vi "Magmapper_Tim.vi"() -> ()   [LabVIEW 2020]
uses:
  Labview_dependencies/locked.vi
  Labview_dependencies/haltnow.vi
  <vilib>/Analysis/NI_AALBase.lvlib
panel:
  out "Lock state":bool
  in  "Centering steps":dbl[](array[numeric])
  in  "Start centering":bool
  in  "Theta abs":dbl
  out "Theta pos":dbl
  in  "Initialisation Theta commands":string[](array[string])=["BASE($$$AXIS$$$)", "BACKLASH(OFF)", "ATYPE=43", "UNITS=16*32", "SPEED=1", "CREEP=.1", "FASTDEC=1", "ACCEL=1", "DECEL=1", "DEFPOS(0)", "WDOG=ON", "BASE(0)"]
  in  "Theta Step":dbl
  in  "Theta End":dbl
  in  "Theta Start":dbl
  out "Theta axis on":bool=TRUE
  in  "Theta rel":dbl
  in  "Z Step":dbl
  in  "Z End":dbl
  in  "Z Start":dbl
  in  "Y Step":dbl
  in  "Y End":dbl
  in  "Y Start":dbl
  in  "X Step":dbl
  in  "X End":dbl
  in  "X Start":dbl
  in  "Clear buffers":bool
  in  "Initialisation XYZ commands":string[](array[string])=["BASE($$$AXIS$$$)", "BACKLASH(OFF)", "ATYPE=43", "UNITS=2560", "SPEED=10", "CREEP=5", "FASTDEC=100", "ACCEL=10", "DECEL=10", "DATUM_IN=$$$AXIS$$$+5", "FS_LIMIT = REP_DIST + 10", "RS_LIMIT = -REP_DIST - 10", "WDOG=ON", "DATUM($$$DATUM$$$)", "ALT_WAIT", "FS_LIMIT=$$$FS$$$", "RS_LIMIT=$$$RS$$$", "BASE(0)"]
  in  "Read grid":bool
  in  "Filename for grid readings":path
  in  "Slope (b)":dbl=1.14189
  in  "Intercept (a)":dbl=-0.010254
  out "message":string="Error messages might appear here."
  in  "Initialise":bool
  in  "Stop movement":bool
  out "Z pos":dbl
  out "Y pos":dbl
  out "X pos":dbl
  in  "Move relative":bool
  in  "Move absolute":bool
  in  "Z rel":dbl
  in  "Y rel":dbl
  in  "X rel":dbl
  in  "Z abs":dbl
  in  "Y abs":dbl
  in  "X abs":dbl
  # "Set field-vs-voltage relationship (B = a + bV)"
  # "Current position"
  # "Move to absolute position"
  # "Move to relative position"
  # "Note: STOP is not yet implemented.\nEither manually stop the VI running \n(usual stop button below menu bar)\nor if urgent turn off the power to the \nmagnet  mapper (red rocker switch)."
  # "Read over grid"
  # "Note: Circular axis should be set  on or off before running the VI, and may not be changed while running."
  # "Greyed items are disabled (not yet implemented)."
  # "List of initialisation commands to feed to the MC 405 controller.  Use ALT_WAIT instead of WAIT IDLE to avoid timeouts.  Commands will be run for each (X,Y,Z) axis, replacing $$$AXIS$$$ with the actual axis, $$$DATUM$$$ with the corresponding datum method, $$$FS$$$ and $$$RS$$$ with the corrsponding limits, each time.   If you change the commands and want to keep them when you close the VI, remember to select the array (whole thing, not just index or individual elements), right click, Data operations, Make Current Value Default."
  # "Move near centre by eye then push start"
  # "Minimum step size is 0.05mm. Micro-stepping down to 0.00625mm is possible but not reccommendded as it not necessarily accurate and may cause excess movement during grid reading"
  # "List of initialisation commands to feed to the MC 405 controller.  Use ALT_WAIT instead of WAIT IDLE to avoid timeouts.  Commands will be run for the Theta axis, replacing $$$AXIS$$$ with the actual axis.   If you change the commands and want to keep them when you close the VI, remember to select the array (whole thing, not just index or individual elements), right click, Data operations, Make Current Value Default."
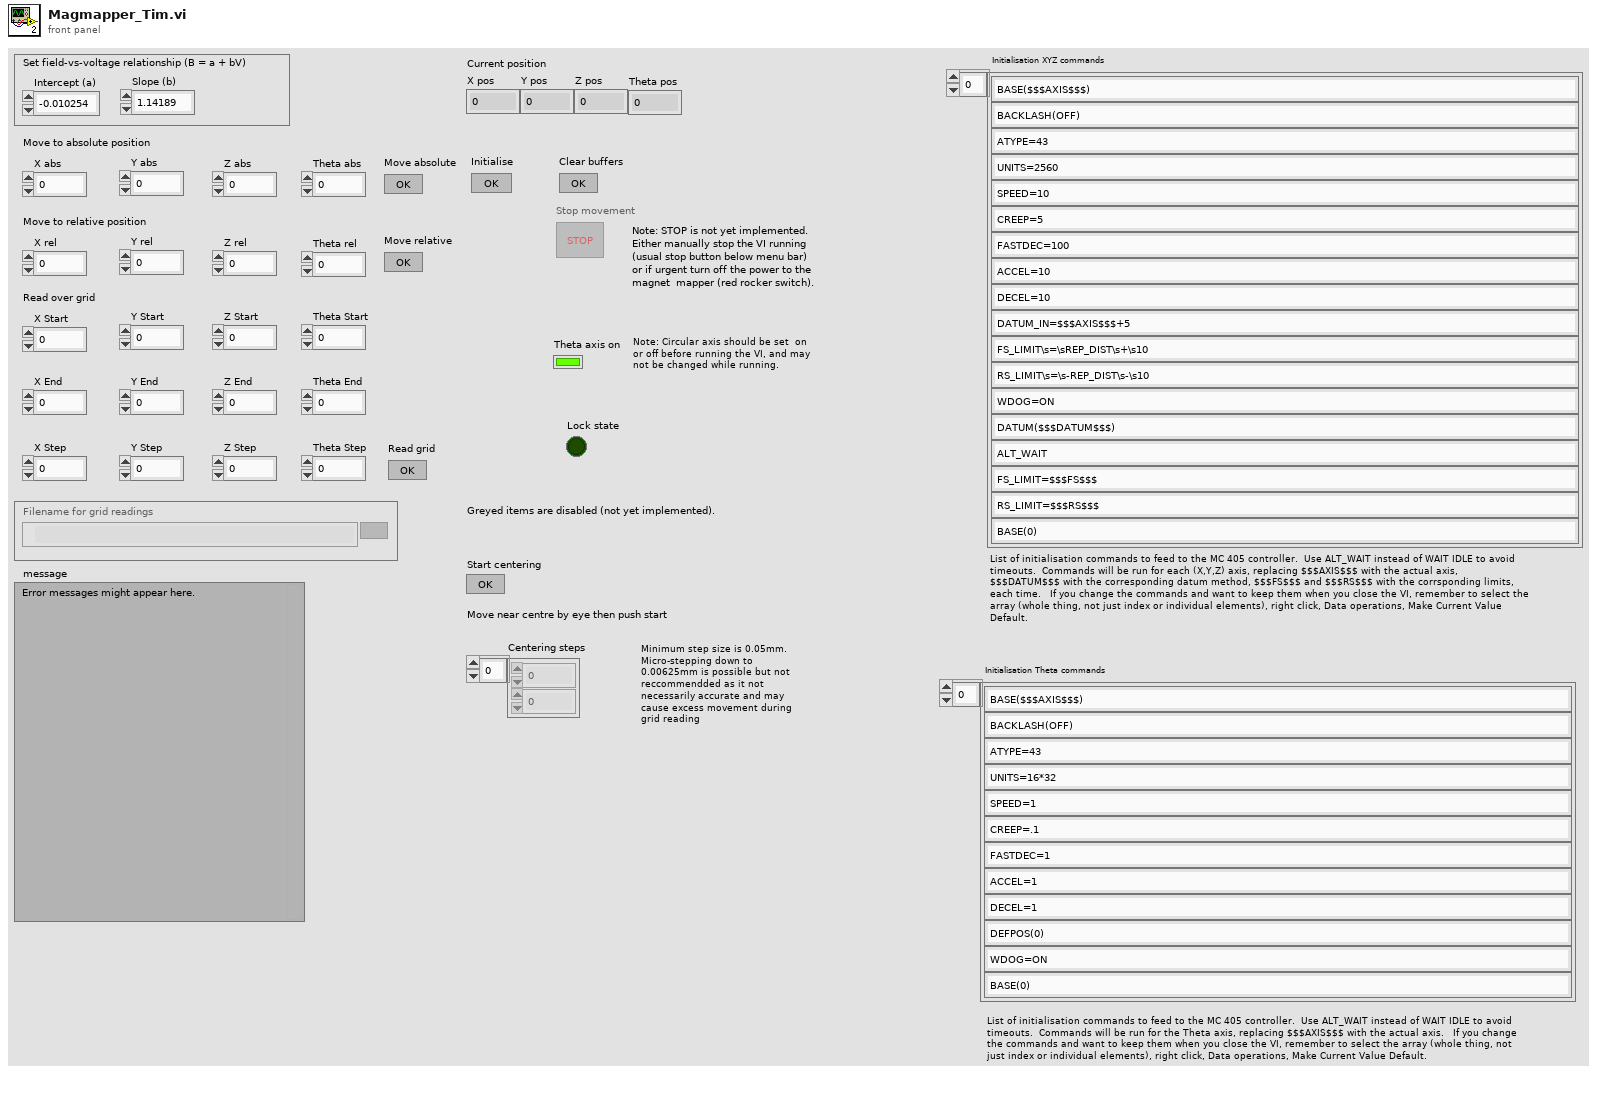
[diagram p1: front panel]
types:
  T1 = enum16{"open", "replace", "create", "open or create", "replace or create", "replace or create with confirmation"}
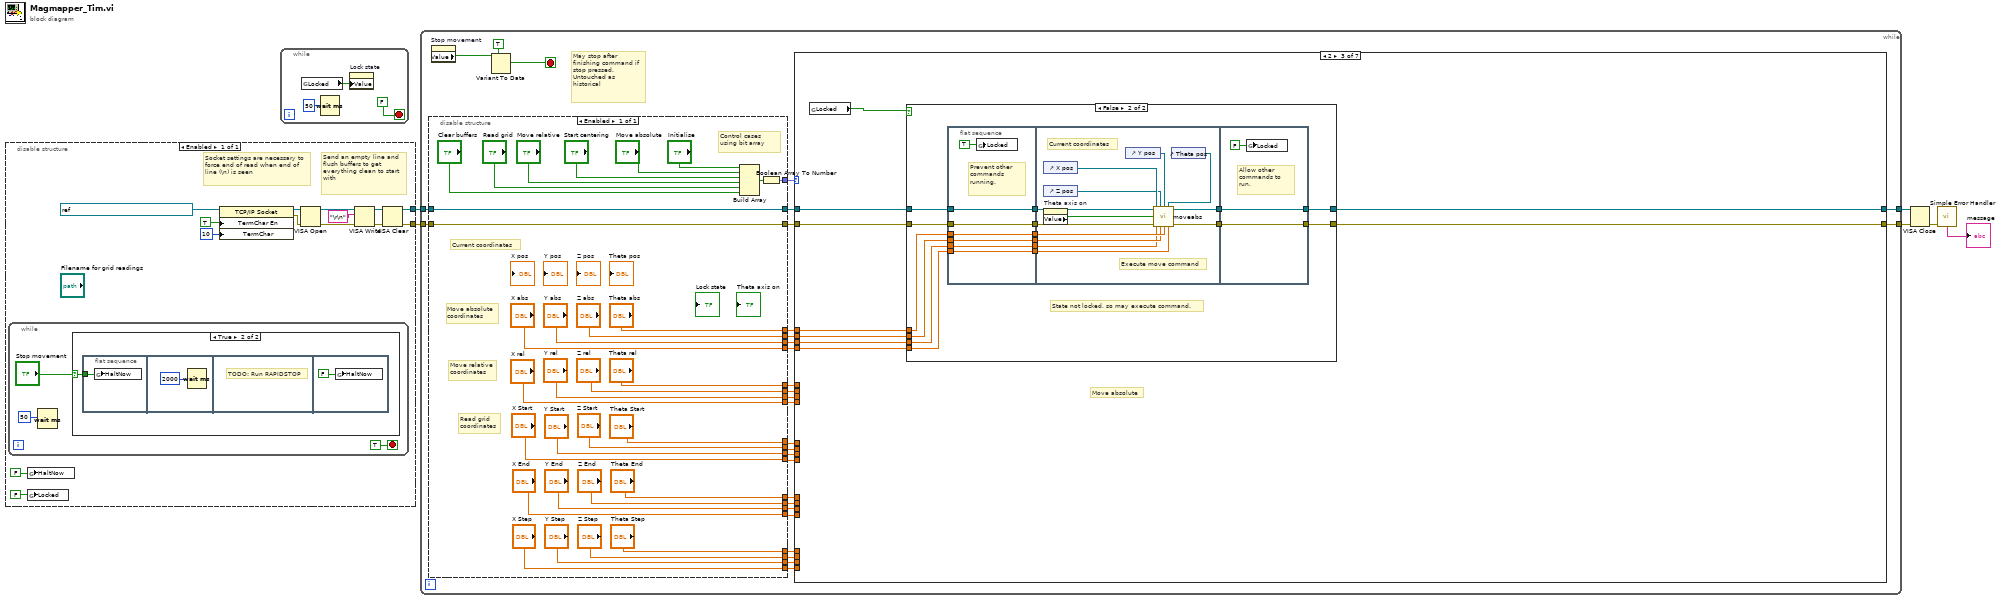
[diagram p0: block diagram]
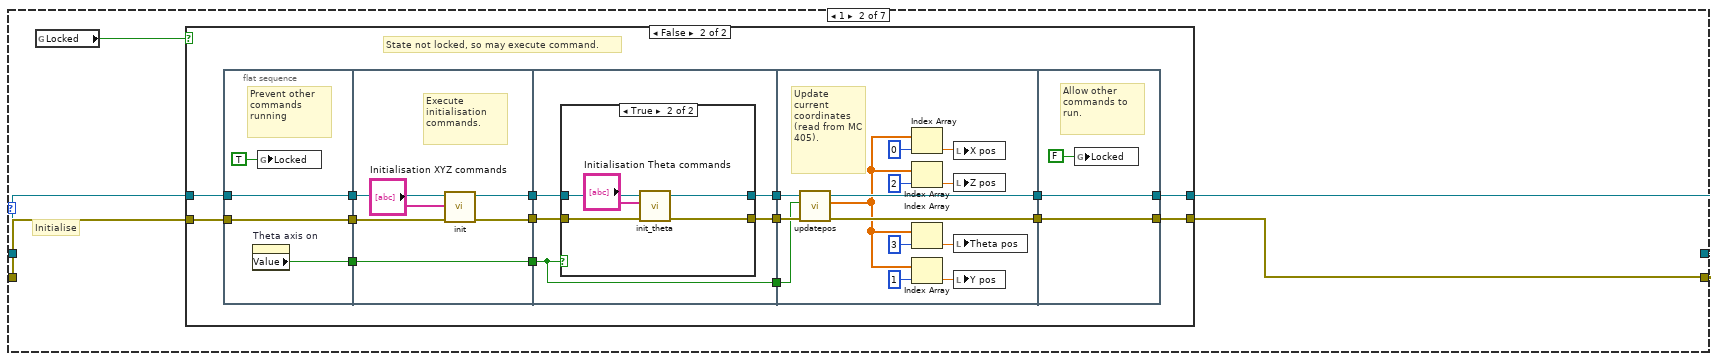
[diagram p4: hidden frame]
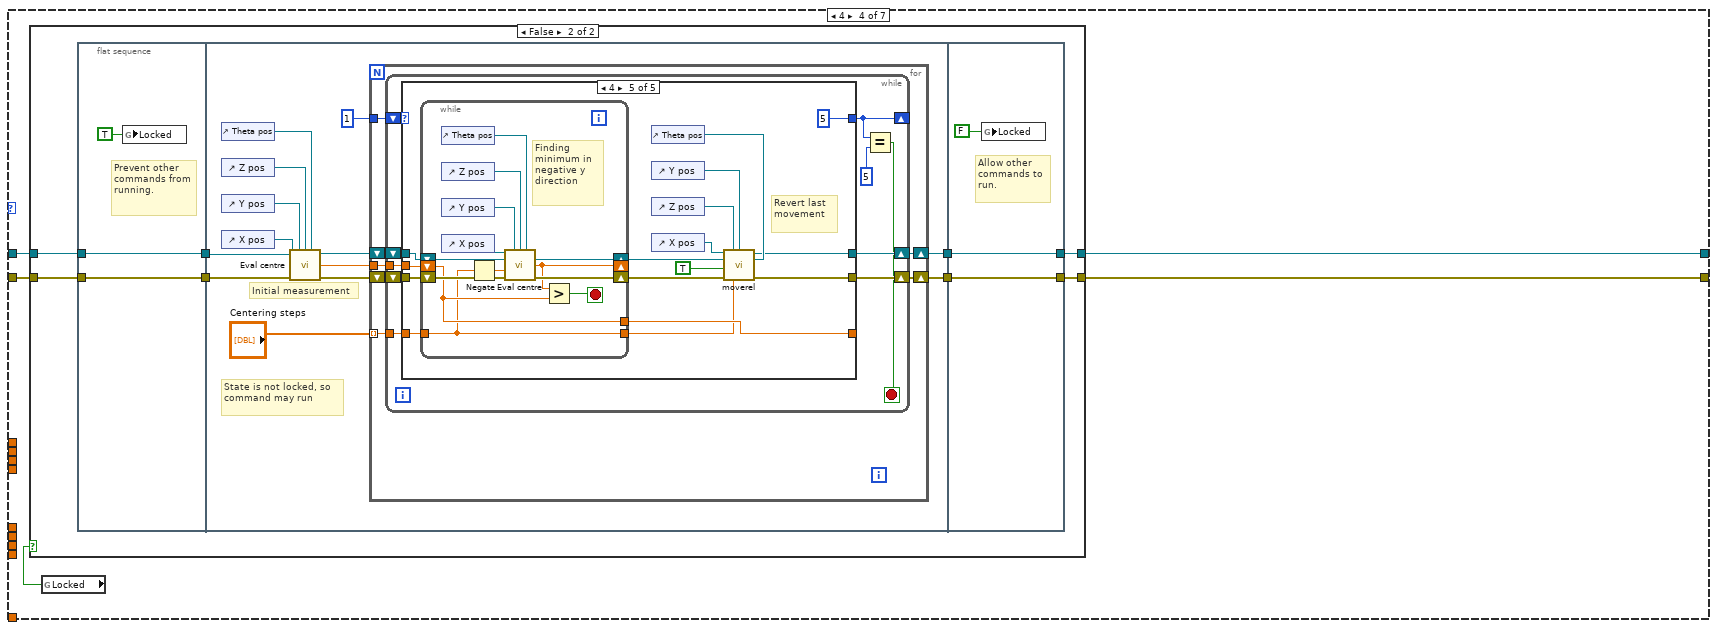
[diagram p8: hidden frame]
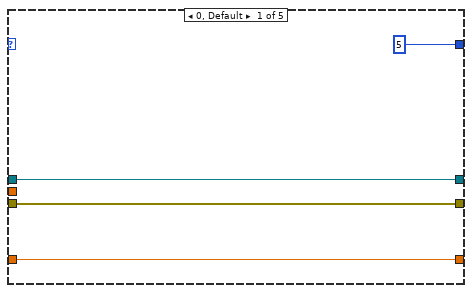
[diagram p10: hidden frame]
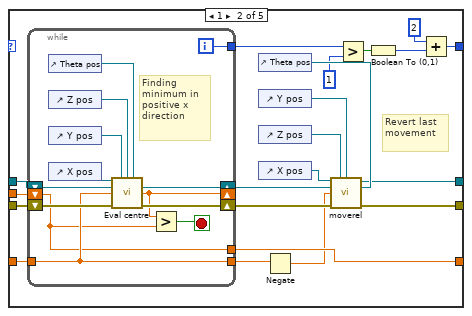
[diagram p11: hidden frame]
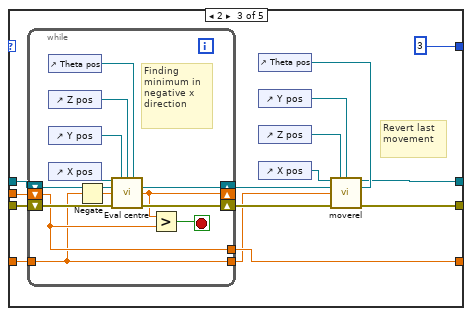
[diagram p12: hidden frame]
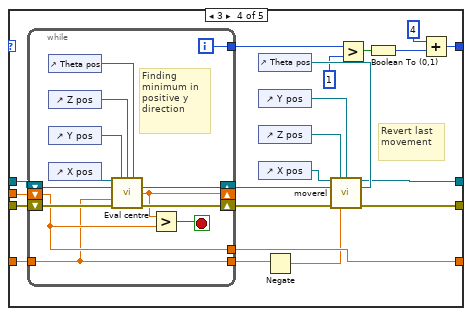
[diagram p13: hidden frame]
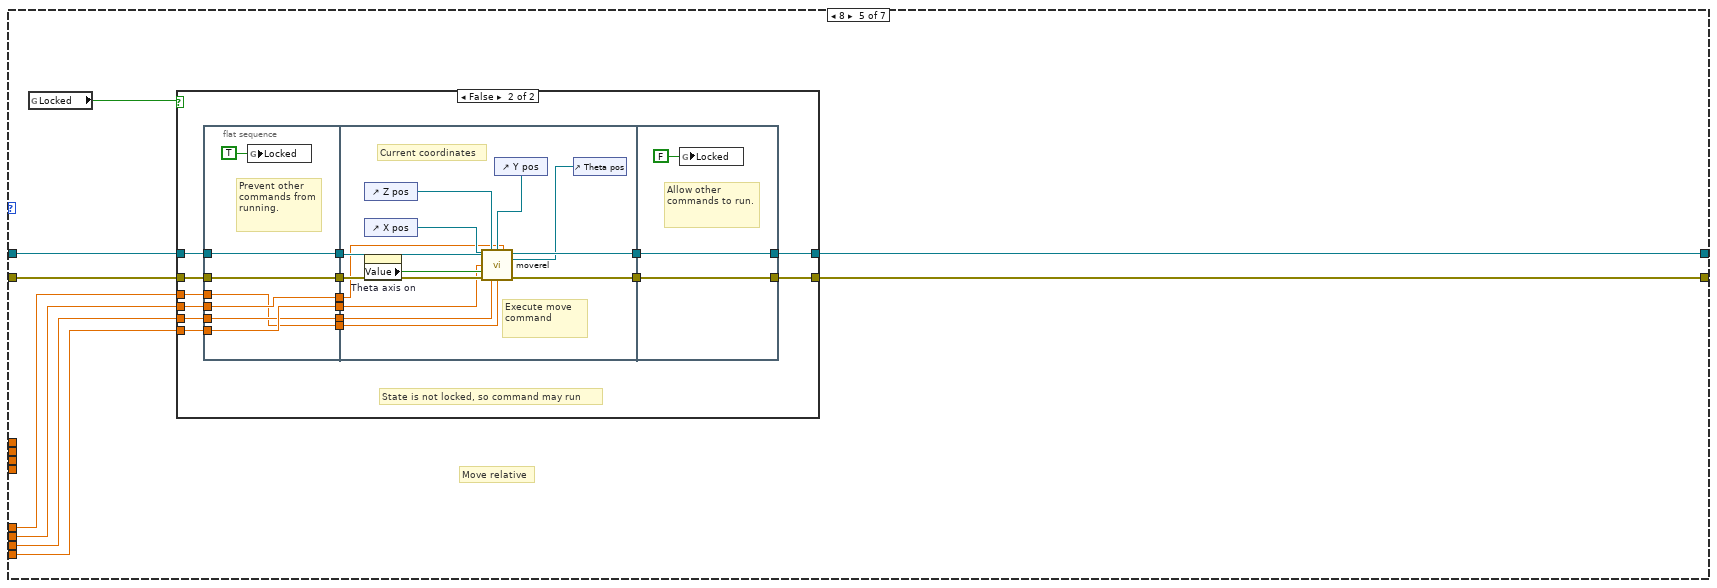
[diagram p14: hidden frame]
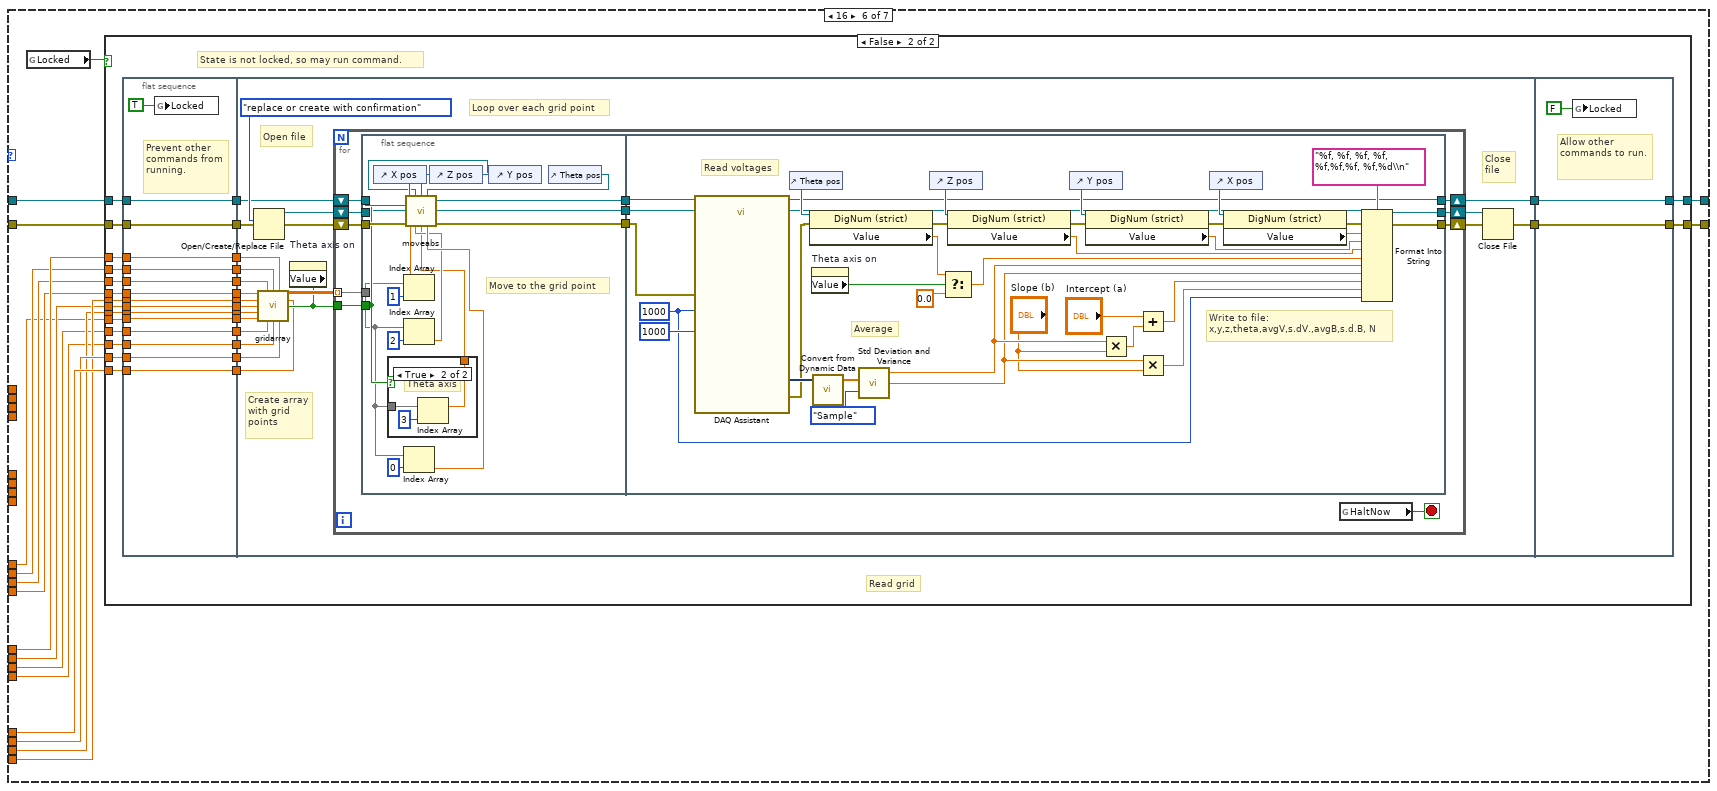
[diagram p16: hidden frame]
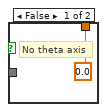
[diagram p18: hidden frame]
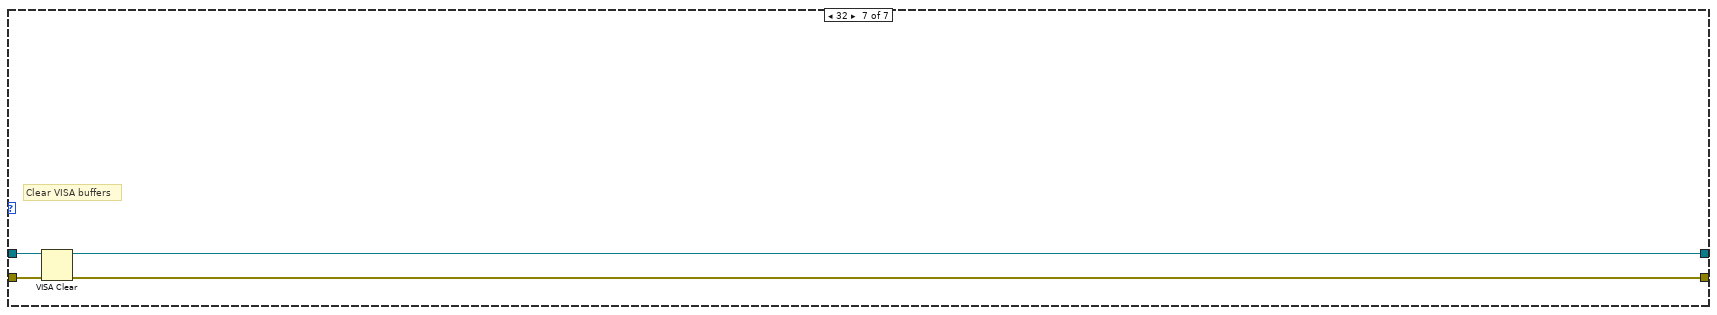
[diagram p19: hidden frame]
diagram:
  n1 = disable-structure shown="Enabled" {
    disable-tunnel: [w19] -> w4
    disable-tunnel: [w18] -> w3
    frame Enabled {
      # "Send an empty line and flush buffers to get everything clean to start with"
      # "Socket settings are necessary to force end of read when end of line (\\n) is seen"
      n2 = while {
        stop <- TRUE stop-if-true
        n3 = Wait (ms)(milliseconds to wait=50) -> ()  [unwired: 1 out]
        n4 = case shown="True" "Stop movement" {
          selector: "Stop movement" -> [_ w24]
          frame False {
          }
          frame True {
            n5 = flat-sequence {
              tunnel: w24 -> [w25]
              frame #0 {
                n6 = global write "haltnow.vi" "HaltNow"(w25) -> ()
              }
              frame #1 {
                n7 = Wait (ms)(milliseconds to wait=u32 2000) -> ()  [unwired: 1 out]
              }
              frame #2 {
                # "TODO: Run RAPIDSTOP"
              }
              frame #3 {
                n8 = global write "haltnow.vi" "HaltNow"(FALSE ("HaltNow")) -> ()
              }
            }
          }
        }
      }
      n9 = global write "haltnow.vi" "HaltNow"(FALSE ("HaltNow")) -> ()
      n10 = global write "locked.vi" "Locked"(FALSE ("Locked")) -> ()
      n11 = property class="TCP/IP Socket"(reference=refnum<visa-resource-name> "TCPIP0::192.168.0.250::23::SOCKET" ("VISA resource name"), "TermChar En"=TRUE ("Message Based Settings:Termination Character Enable"), "TermChar"=u8 10 ("Message Based Settings:Termination Character")) -> (reference out=w13:refnum<visa-resource-name>, error out=w12:errorcluster)  [unwired: 1 in]
      n12 = VISA Open(error in (no error)=w12, VISA resource name=w13) -> (VISA resource name=w10:refnum<visa-resource-name>, error out=w9:errorcluster)  [unwired: 3 in]
      n13 = VISA Write(VISA resource name=w10, write buffer="\r\n", error in (no error)=w9) -> (VISA resource name out=w8:refnum<visa-resource-name>, error out=w7:errorcluster)  [unwired: 1 out]
      n14 = VISA Clear(VISA resource name=w8, error in (no error)=w7) -> (VISA resource name out=w19:refnum<visa-resource-name>, error out=w18:errorcluster)
    }
  }
  n15 = while {
    stop <- FALSE stop-if-true
    n16 = global read "locked.vi" "Locked"() -> (w30:bool)
    n17 = Wait (ms)(milliseconds to wait=50) -> ()  [unwired: 1 out]
    n18 = property on="Lock state" class="Bool (strict)"("Value"=w30) -> ()  [unwired: 2 in, 2 out]
  }
  n19 = while {
    tunnel: w4 -> [w32]
    tunnel: w3 -> [w33]
    tunnel: [w59] -> w1
    tunnel: [w58] -> w2
    stop <- w35 stop-if-true
    # "May stop after finishing command if stop pressed. Untouched as historical"
    n20 = disable-structure shown="Enabled" {
      disable-tunnel: [w90] -> w60
      disable-tunnel: ["Theta Step"] -> w57
      disable-tunnel: ["Theta abs"] -> w56
      disable-tunnel: ["Theta End"] -> w55
      disable-tunnel: ["Theta Start"] -> w54
      disable-tunnel: ["Theta rel"] -> w53
      disable-tunnel: ["Z Step"] -> w52
      disable-tunnel: ["Z End"] -> w51
      disable-tunnel: ["Z Start"] -> w50
      disable-tunnel: ["Y Step"] -> w49
      disable-tunnel: ["Y End"] -> w48
      disable-tunnel: ["Y Start"] -> w47
      disable-tunnel: ["X Step"] -> w46
      disable-tunnel: ["X End"] -> w45
      disable-tunnel: ["X Start"] -> w44
      disable-tunnel: ["Z rel"] -> w43
      disable-tunnel: ["Y rel"] -> w42
      disable-tunnel: ["X rel"] -> w41
      disable-tunnel: ["Z abs"] -> w40
      disable-tunnel: ["Y abs"] -> w39
      disable-tunnel: ["X abs"] -> w38
      disable-tunnel: [w62] -> w34
      disable-tunnel: w33 -> [w62]
      disable-tunnel: w32 -> [w61]
      disable-tunnel: [w61] -> w31
      frame Enabled {
        # "Current coordinates"
        # "Move absolute\ncoordinates"
        # "Move relative\ncoordinates"
        # "Read grid\ncoordinates"
        # "Control cases using bit array"
        n21 = Build Array("Initialise", "Move absolute", "Start centering", "Move relative", "Read grid", "Clear buffers") -> (w86:bool[])
        n22 = Boolean Array To Number(Boolean array=w86) -> (number=w90:fxp<+,8,8>)
      }
    }
    n23 = property on="Stop movement" class="Bool (strict)"() -> ("Value"=w37:bool)  [unwired: 2 in, 2 out]
    n24 = Variant To Data(type=TRUE, Variant=w37) -> (data=w35:bool)  [unwired: 1 in, 1 out]
    n25 = case shown="2" w60 {
      tunnel: w34 -> [w92 w96 w162 w206 w392 w446 w596]
      tunnel: w31 -> [w91 w95 w161 w207 w385 w448 w597]
      tunnel: w38 -> [_ _ w160 _ _ _ _]
      tunnel: w39 -> [_ _ w159 _ _ _ _]
      tunnel: w40 -> [_ _ w158 _ _ _ _]
      tunnel: w41 -> [_ _ _ _ w390 _ _]
      tunnel: w42 -> [_ _ _ _ w389 _ _]
      tunnel: w43 -> [_ _ _ _ w388 _ _]
      tunnel: [w91 w93 w155 w205 w386 w449 w595] -> w59
      tunnel: [w92 w94 w156 w204 w387 w447 w594] -> w58
      tunnel: w50 -> [_ _ _ _ _ w435 _]
      tunnel: w47 -> [_ _ _ _ _ w436 _]
      tunnel: w44 -> [_ _ _ _ _ w437 _]
      tunnel: w46 -> [_ _ _ _ _ w443 _]
      tunnel: w51 -> [_ _ _ _ _ w441 _]
      tunnel: w49 -> [_ _ _ _ _ w442 _]
      tunnel: w48 -> [_ _ _ _ _ w439 _]
      tunnel: w45 -> [_ _ _ _ _ w438 _]
      tunnel: w52 -> [_ _ _ _ _ w444 _]
      tunnel: w56 -> [_ _ w154 _ _ _ _]
      tunnel: w53 -> [_ _ _ _ w384 _ _]
      tunnel: w55 -> [_ _ _ _ _ w440 _]
      tunnel: w54 -> [_ _ _ _ _ w434 _]
      tunnel: w57 -> [_ _ _ _ _ w445 _]
      frame 0, Default {
        # "No command chosen.  Do nothing."
      }
      frame 1 {
        # "Initialise"
        n26 = global read "locked.vi" "Locked"() -> (w97:bool)
        n27 = case shown="False" w97 {
          tunnel: w96 -> [w98 w114]
          tunnel: w95 -> [w99 w113]
          tunnel: [w99 w108] -> w93
          tunnel: [w98 w107] -> w94
          frame True {
            # "State locked, so don't execute command."
          }
          frame False {
            # "State not locked, so may execute command."
            n28 = flat-sequence {
              tunnel: w113 -> [w117]
              tunnel: w114 -> [w118]
              tunnel: [w118] -> w112
              tunnel: [w117] -> w111
              tunnel: [w115] -> w101
              tunnel: w112 -> [w124]
              tunnel: w111 -> [w123]
              tunnel: [w121] -> w106
              tunnel: [w120] -> w104
              tunnel: [w119] -> w102
              tunnel: w101 -> [w119]
              tunnel: w106 -> [w126]
              tunnel: [w129] -> w105
              tunnel: w104 -> [w127]
              tunnel: [w128] -> w103
              tunnel: w102 -> [w125]
              tunnel: [w125] -> w100
              tunnel: w105 -> [w145]
              tunnel: [w144] -> w110
              tunnel: w103 -> [w147]
              tunnel: [w146] -> w109
              tunnel: w100 -> [w137]
              tunnel: [w152] -> w107
              tunnel: w110 -> [w152]
              tunnel: [w151] -> w108
              tunnel: w109 -> [w151]
              frame #0 {
                # "Prevent other commands running"
                n29 = property on="Theta axis on" class="Bool (strict)"() -> ("Value"=w115:bool)  [unwired: 2 in, 2 out]
                n30 = global write "locked.vi" "Locked"(TRUE ("Locked")) -> ()
              }
              frame #1 {
                # "Execute initialisation commands."
                n31 = call "init.vi"("error in (no error)"=w124, "Commands to run"="Initialisation XYZ commands", "VISA Refnum in"=w123) -> ("error out"=w121:errorcluster, "VISA Refnum out"=w120:refnum<visa-resource-name>)  [unwired: 7 in]
              }
              frame #2 {
                n32 = case shown="True" w125 {
                  tunnel: [w130 w136] -> w129
                  tunnel: [w131 w135] -> w128
                  tunnel: w127 -> [w131 w134]
                  tunnel: w126 -> [w130 w133]
                  frame False {
                  }
                  frame True {
                    n33 = call "init_theta.vi"("error in (no error)"=w133, "Commands to run"="Initialisation Theta commands", "VISA Refnum in"=w134) -> ("error out"=w136:errorcluster, "VISA Refnum out"=w135:refnum<visa-resource-name>)  [unwired: 7 in]
                  }
                }
              }
              frame #3 {
                # "Update current coordinates (read from MC 405)."
                n34 = call "updatepos.vi"("error in (no error)"=w145, "Theta enabled"=w137, "VISA Refnum in"=w147) -> ("error out"=w144:errorcluster, "PosArray"=w139:dbl[], "VISA Refnum out"=w146:refnum<visa-resource-name>)  [unwired: 6 in]
                n35 = Index Array(array=w139, index=0) -> (element=w143:dbl)
                n36 = Index Array(array=w139, index=2) -> (element=w141:dbl)
                n37 = Index Array(array=w139, index=3) -> (element=w138:dbl)
                n38 = Index Array(array=w139, index=1) -> (element=w142:dbl)
                n39 = local write "X pos"(w143) -> ()
                n40 = local write "Z pos"(w141) -> ()
                n41 = local write "Theta pos"(w138) -> ()
                n42 = local write "Y pos"(w142) -> ()
              }
              frame #4 {
                # "Allow other commands to run."
                n43 = global write "locked.vi" "Locked"(FALSE ("Locked")) -> ()
              }
            }
          }
        }
      }
      frame 2 {
        # "Move absolute"
        n44 = global read "locked.vi" "Locked"() -> (w157:bool)
        n45 = case shown="False" w157 {
          tunnel: w162 -> [w163 w180]
          tunnel: w161 -> [w164 w179]
          tunnel: w160 -> [_ w169]
          tunnel: w159 -> [_ w170]
          tunnel: w158 -> [_ w171]
          tunnel: [w164 w174] -> w155
          tunnel: [w163 w173] -> w156
          tunnel: w154 -> [_ w172]
          frame True {
            # "State locked, so don't execute command."
          }
          frame False {
            # "State not locked, so may execute command."
            n46 = flat-sequence {
              tunnel: w179 -> [w186]
              tunnel: w180 -> [w187]
              tunnel: [w187] -> w178
              tunnel: [w186] -> w177
              tunnel: w172 -> [w184]
              tunnel: w171 -> [w183]
              tunnel: w170 -> [w182]
              tunnel: w169 -> [w181]
              tunnel: [w184] -> w168
              tunnel: [w183] -> w167
              tunnel: [w182] -> w166
              tunnel: [w181] -> w165
              tunnel: w178 -> [w200]
              tunnel: w177 -> [w199]
              tunnel: [w198] -> w176
              tunnel: [w197] -> w175
              tunnel: w168 -> [w191]
              tunnel: w167 -> [w190]
              tunnel: w166 -> [w189]
              tunnel: w165 -> [w188]
              tunnel: [w201] -> w173
              tunnel: [w202] -> w174
              tunnel: w176 -> [w202]
              tunnel: w175 -> [w201]
              frame #0 {
                # "Prevent other commands running."
                n47 = global write "locked.vi" "Locked"(TRUE ("Locked")) -> ()
              }
              frame #1 {
                # "Execute move command"
                # "Current coordinates"
                n48 = control-ref of="X pos"() -> (w196:refnum<vi>)
                n49 = control-ref of="Z pos"() -> (w194:refnum<vi>)
                n50 = property on="Theta axis on" class="Bool (strict)"() -> ("Value"=w193:bool)  [unwired: 2 in, 2 out]
                n51 = control-ref of="Y pos"() -> (w195:refnum<vi>)
                n52 = control-ref of="Theta pos"() -> (w192:refnum<vi>)
                n53 = call "moveabs.vi"("Xpos"=w196, "ZPos"=w194, "YPos"=w195, "ThetaPos"=w192, "VISA resource name"=w199, "Theta on"=w193, "Y"=w189, "error in (no error)"=w200, "Z"=w190, "Theta"=w191, "X"=w188) -> ("VISA Refnum out"=w198:refnum<visa-resource-name>, "error out"=w197:errorcluster)  [unwired: 3 in]
              }
              frame #2 {
                # "Allow other commands to run."
                n54 = global write "locked.vi" "Locked"(FALSE ("Locked")) -> ()
              }
            }
          }
        }
      }
      frame 4 {
        n55 = global read "locked.vi" "Locked"() -> (w208:bool)
        n56 = case shown="False" w208 {
          tunnel: [w209 w211] -> w204
          tunnel: [w210 w212] -> w205
          tunnel: w207 -> [w210 w218]
          tunnel: w206 -> [w209 w217]
          frame True {
            # "State is locked.  Do not run command."
          }
          frame False {
            n57 = flat-sequence {
              tunnel: w217 -> [w220]
              tunnel: w218 -> [w221]
              tunnel: [w221] -> w216
              tunnel: [w220] -> w215
              tunnel: w216 -> [w227]
              tunnel: w215 -> [w226]
              tunnel: [w225] -> w214
              tunnel: [w224] -> w213
              tunnel: w214 -> [w382]
              tunnel: w213 -> [w381]
              tunnel: [w382] -> w212
              tunnel: [w381] -> w211
              frame #0 {
                # "Prevent other commands from running."
                n58 = global write "locked.vi" "Locked"(TRUE ("Locked")) -> ()
              }
              frame #1 {
                # "Initial measurement"
                # "State is not locked, so command may run"
                n59 = control-ref of="Theta pos"() -> (w229:refnum<vi>)
                n60 = control-ref of="Z pos"() -> (w230:refnum<vi>)
                n61 = control-ref of="Y pos"() -> (w231:refnum<vi>)
                n62 = control-ref of="X pos"() -> (w232:refnum<vi>)
                n63 = call "Eval centre.vi"("Xpos"=w232, "Ypos"=w231, "Zpos"=w230, "Thetapos"=w229, "VISA resource name"=w227, "error in (no error)"=w226) -> ("VISA Refnum out"=w234:refnum<visa-resource-name>, "Difference"=w228:dbl, "error out"=w233:errorcluster)  [unwired: 4 in, 3 out]
                n64 = for {
                  tunnel: "Centering steps" -> [w238] mode=indexing
                  tunnel: w228 -> [w239]
                  shift-right: [w237] -> w225
                  shift-left: w234 -> [w241]
                  shift-right: [w236] -> w224
                  shift-left: w233 -> [w240]
                  tunnel: 1 -> [w235]
                  n65 = while {
                    tunnel: w239 -> [w249]
                    tunnel: w238 -> [w248]
                    shift-right: [w246] -> w237
                    shift-left: w241 -> [w251]
                    shift-right: [w245] -> w236
                    shift-left: w240 -> [w250]
                    shift-right: [w244] -> _
                    shift-left: w235 -> [w247]
                    stop <- w242 stop-if-true
                    n66 = case shown="4" w247 {
                      tunnel: w251 -> [w255 w272 w300 w334 w363]
                      tunnel: [w255 w271 w299 w333 w362] -> w246
                      tunnel: [w254 w270 w298 w332 w361] -> w245
                      tunnel: w250 -> [w254 w269 w297 w331 w360]
                      tunnel: w248 -> [w253 w266 w294 w328 w357]
                      tunnel: w249 -> [_ w265 w293 w327 w356]
                      tunnel: [w253 w264 w292 w326 w355] -> _
                      tunnel: [5 w259 3 w322 5] -> w244
                      frame 0, Default {
                      }
                      frame 1 {
                        # "Revert last movement"
                        n67 = while {
                          shift-right: [w286] -> w268
                          shift-left: w269 -> [w287]
                          shift-right: [w288] -> w267
                          shift-left: w272 -> [w289]
                          tunnel: w266 -> [w280]
                          tunnel: [w280] -> w263
                          shift-right: [w277] -> _
                          shift-left: w265 -> [w279]
                          tunnel: [w279] -> w264
                          tunnel: [w278] -> w261
                          i -> [w278]
                          stop <- w281 stop-if-true
                          # "Finding minimum in positive x direction"
                          n68 = control-ref of="Theta pos"() -> (w282:refnum<vi>)
                          n69 = control-ref of="Z pos"() -> (w283:refnum<vi>)
                          n70 = control-ref of="Y pos"() -> (w284:refnum<vi>)
                          n71 = control-ref of="X pos"() -> (w285:refnum<vi>)
                          n72 = call "Eval centre.vi"("Xpos"=w285, "Ypos"=w284, "Zpos"=w283, "Thetapos"=w282, "VISA resource name"=w289, "X inc"=w280, "error in (no error)"=w287) -> ("VISA Refnum out"=w288:refnum<visa-resource-name>, "Difference"=w277:dbl, "error out"=w286:errorcluster)  [unwired: 3 in, 3 out]
                          n73 = Greater?(x=w277, y=w279) -> (0:w281:bool)
                        }
                        n74 = control-ref of="Theta pos"() -> (w276:refnum<vi>)
                        n75 = control-ref of="Y pos"() -> (w274:refnum<vi>)
                        n76 = control-ref of="Z pos"() -> (w273:refnum<vi>)
                        n77 = control-ref of="X pos"() -> (w275:refnum<vi>)
                        n78 = Negate(x=w263) -> (-x=w262:dbl)
                        n79 = call "moverel.vi"("Xpos"=w275, "Zpos"=w273, "Ypos"=w274, "VISA resource name"=w267, "Thetapos"=w276, "X increment"=w262, "error in (no error)"=w268) -> ("VISA Refnum out"=w271:refnum<visa-resource-name>, "error out"=w270:errorcluster)  [unwired: 7 in]
                        n80 = Greater?(x=w261, y=1) -> (0:w258:bool)
                        n81 = Boolean To (0,1)(Boolean=w258) -> (0, 1=w256:i16)
                        n82 = Add(x=2, y=w256) -> (x+y=w259:i32)
                      }
                      frame 2 {
                        # "Revert last movement"
                        n83 = while {
                          shift-right: [w314] -> w296
                          shift-left: w297 -> [w315]
                          shift-right: [w316] -> w295
                          shift-left: w300 -> [w317]
                          tunnel: w294 -> [w306]
                          tunnel: [w306] -> w291
                          shift-right: [w307] -> _
                          shift-left: w293 -> [w308]
                          tunnel: [w308] -> w292
                          stop <- w309 stop-if-true
                          # "Finding minimum in negative x direction"
                          n84 = control-ref of="Theta pos"() -> (w310:refnum<vi>)
                          n85 = control-ref of="Z pos"() -> (w311:refnum<vi>)
                          n86 = control-ref of="Y pos"() -> (w312:refnum<vi>)
                          n87 = control-ref of="X pos"() -> (w313:refnum<vi>)
                          n88 = Negate(x=w306) -> (-x=w305:dbl)
                          n89 = call "Eval centre.vi"("Xpos"=w313, "Ypos"=w312, "Zpos"=w311, "Thetapos"=w310, "VISA resource name"=w317, "X inc"=w305, "error in (no error)"=w315) -> ("VISA Refnum out"=w316:refnum<visa-resource-name>, "Difference"=w307:dbl, "error out"=w314:errorcluster)  [unwired: 3 in, 3 out]
                          n90 = Greater?(x=w307, y=w308) -> (0:w309:bool)
                        }
                        n91 = control-ref of="Theta pos"() -> (w304:refnum<vi>)
                        n92 = control-ref of="Y pos"() -> (w302:refnum<vi>)
                        n93 = control-ref of="Z pos"() -> (w301:refnum<vi>)
                        n94 = control-ref of="X pos"() -> (w303:refnum<vi>)
                        n95 = call "moverel.vi"("Xpos"=w303, "Zpos"=w301, "Ypos"=w302, "VISA resource name"=w295, "Thetapos"=w304, "X increment"=w291, "error in (no error)"=w296) -> ("VISA Refnum out"=w299:refnum<visa-resource-name>, "error out"=w298:errorcluster)  [unwired: 7 in]
                      }
                      frame 3 {
                        # "Revert last movement"
                        n96 = while {
                          shift-right: [w348] -> w330
                          shift-left: w331 -> [w349]
                          shift-right: [w350] -> w329
                          shift-left: w334 -> [w351]
                          tunnel: w328 -> [w339]
                          tunnel: [w339] -> w325
                          shift-right: [w340] -> _
                          shift-left: w327 -> [w342]
                          tunnel: [w342] -> w326
                          tunnel: [w341] -> w324
                          i -> [w341]
                          stop <- w343 stop-if-true
                          # "Finding minimum in positive y direction"
                          n97 = control-ref of="Theta pos"() -> (w344:refnum<vi>)
                          n98 = control-ref of="Z pos"() -> (w345:refnum<vi>)
                          n99 = control-ref of="Y pos"() -> (w346:refnum<vi>)
                          n100 = control-ref of="X pos"() -> (w347:refnum<vi>)
                          n101 = call "Eval centre.vi"("Xpos"=w347, "Ypos"=w346, "Zpos"=w345, "Thetapos"=w344, "VISA resource name"=w351, "Y inc"=w339, "error in (no error)"=w349) -> ("VISA Refnum out"=w350:refnum<visa-resource-name>, "Difference"=w340:dbl, "error out"=w348:errorcluster)  [unwired: 3 in, 3 out]
                          n102 = Greater?(x=w340, y=w342) -> (0:w343:bool)
                        }
                        n103 = control-ref of="Theta pos"() -> (w338:refnum<vi>)
                        n104 = control-ref of="Y pos"() -> (w336:refnum<vi>)
                        n105 = control-ref of="Z pos"() -> (w335:refnum<vi>)
                        n106 = control-ref of="X pos"() -> (w337:refnum<vi>)
                        n107 = Negate(x=w325) -> (-x=w320:dbl)
                        n108 = call "moverel.vi"("Xpos"=w337, "Zpos"=w335, "Ypos"=w336, "VISA resource name"=w329, "Thetapos"=w338, "error in (no error)"=w330, "Y increment"=w320) -> ("VISA Refnum out"=w333:refnum<visa-resource-name>, "error out"=w332:errorcluster)  [unwired: 7 in]
                        n109 = Greater?(x=w324, y=1) -> (0:w321:bool)
                        n110 = Boolean To (0,1)(Boolean=w321) -> (0, 1=w319:i16)
                        n111 = Add(x=4, y=w319) -> (x+y=w322:i32)
                      }
                      frame 4 {
                        # "Revert last movement"
                        n112 = while {
                          shift-right: [w377] -> w359
                          shift-left: w360 -> [w378]
                          shift-right: [w379] -> w358
                          shift-left: w363 -> [w380]
                          tunnel: w357 -> [w368]
                          tunnel: [w368] -> w354
                          shift-right: [w370] -> _
                          shift-left: w356 -> [w371]
                          tunnel: [w371] -> w355
                          stop <- w372 stop-if-true
                          # "Finding minimum in negative y direction"
                          n113 = control-ref of="Theta pos"() -> (w373:refnum<vi>)
                          n114 = control-ref of="Z pos"() -> (w374:refnum<vi>)
                          n115 = control-ref of="Y pos"() -> (w375:refnum<vi>)
                          n116 = control-ref of="X pos"() -> (w376:refnum<vi>)
                          n117 = Negate(x=w368) -> (-x=w369:dbl)
                          n118 = call "Eval centre.vi"("Xpos"=w376, "Ypos"=w375, "Zpos"=w374, "Thetapos"=w373, "VISA resource name"=w380, "Y inc"=w369, "error in (no error)"=w378) -> ("VISA Refnum out"=w379:refnum<visa-resource-name>, "Difference"=w370:dbl, "error out"=w377:errorcluster)  [unwired: 3 in, 3 out]
                          n119 = Greater?(x=w370, y=w371) -> (0:w372:bool)
                        }
                        n120 = control-ref of="Theta pos"() -> (w367:refnum<vi>)
                        n121 = control-ref of="Y pos"() -> (w365:refnum<vi>)
                        n122 = control-ref of="Z pos"() -> (w364:refnum<vi>)
                        n123 = control-ref of="X pos"() -> (w366:refnum<vi>)
                        n124 = call "moverel.vi"("Xpos"=w366, "Zpos"=w364, "Ypos"=w365, "VISA resource name"=w358, "Thetapos"=w367, "Theta on"=TRUE, "error in (no error)"=w359, "Y increment"=w354) -> ("VISA Refnum out"=w362:refnum<visa-resource-name>, "error out"=w361:errorcluster)  [unwired: 6 in]
                      }
                    }
                    n125 = Equal?(x=w244, y=5) -> (x = y?=w242:bool)
                  }
                }
              }
              frame #2 {
                # "Allow other commands to run."
                n126 = global write "locked.vi" "Locked"(FALSE ("Locked")) -> ()
              }
            }
          }
        }
      }
      frame 8 {
        # "Move relative"
        n127 = global read "locked.vi" "Locked"() -> (w391:bool)
        n128 = case shown="False" w391 {
          tunnel: w392 -> [w393 w410]
          tunnel: w385 -> [w394 w409]
          tunnel: w390 -> [_ w401]
          tunnel: w389 -> [_ w400]
          tunnel: w388 -> [_ w398]
          tunnel: [w393 w404] -> w387
          tunnel: [w394 w403] -> w386
          tunnel: w384 -> [_ w396]
          frame True {
            # "State is locked.  Do not run command."
          }
          frame False {
            # "State is not locked, so command may run"
            n129 = flat-sequence {
              tunnel: w409 -> [w416]
              tunnel: w410 -> [w417]
              tunnel: [w417] -> w408
              tunnel: [w416] -> w407
              tunnel: [w414] -> w402
              tunnel: w401 -> [w414]
              tunnel: w400 -> [w413]
              tunnel: [w413] -> w399
              tunnel: w398 -> [w412]
              tunnel: [w412] -> w397
              tunnel: w396 -> [w411]
              tunnel: [w411] -> w395
              tunnel: w408 -> [w430]
              tunnel: w407 -> [w429]
              tunnel: [w428] -> w406
              tunnel: [w427] -> w405
              tunnel: w402 -> [w421]
              tunnel: w399 -> [w420]
              tunnel: w397 -> [w419]
              tunnel: w395 -> [w418]
              tunnel: w406 -> [w431]
              tunnel: w405 -> [w432]
              tunnel: [w432] -> w404
              tunnel: [w431] -> w403
              frame #0 {
                # "Prevent other commands from running."
                n130 = global write "locked.vi" "Locked"(TRUE ("Locked")) -> ()
              }
              frame #1 {
                # "Execute move command"
                # "Current coordinates"
                n131 = control-ref of="Z pos"() -> (w424:refnum<vi>)
                n132 = control-ref of="X pos"() -> (w425:refnum<vi>)
                n133 = property on="Theta axis on" class="Bool (strict)"() -> ("Value"=w426:bool)  [unwired: 2 in, 2 out]
                n134 = control-ref of="Y pos"() -> (w423:refnum<vi>)
                n135 = control-ref of="Theta pos"() -> (w422:refnum<vi>)
                n136 = call "moverel.vi"("Xpos"=w425, "Zpos"=w424, "Ypos"=w423, "Z increment"=w419, "VISA resource name"=w429, "Thetapos"=w422, "X increment"=w421, "Theta on"=w426, "error in (no error)"=w430, "Y increment"=w420, "Theta inc"=w418) -> ("VISA Refnum out"=w428:refnum<visa-resource-name>, "error out"=w427:errorcluster)  [unwired: 3 in]
              }
              frame #2 {
                # "Allow other commands to run."
                n137 = global write "locked.vi" "Locked"(FALSE ("Locked")) -> ()
              }
            }
          }
        }
      }
      frame 16 {
        n138 = global read "locked.vi" "Locked"() -> (w450:bool)
        n139 = case shown="False" w450 {
          tunnel: [w452 w482] -> w449
          tunnel: w448 -> [w452 w454]
          tunnel: [w451 w481] -> w447
          tunnel: w446 -> [w451 w478]
          tunnel: w445 -> [_ w477]
          tunnel: w444 -> [_ w476]
          tunnel: w443 -> [_ w473]
          tunnel: w442 -> [_ w471]
          tunnel: w441 -> [_ w470]
          tunnel: w440 -> [_ w468]
          tunnel: w439 -> [_ w466]
          tunnel: w438 -> [_ w464]
          tunnel: w437 -> [_ w462]
          tunnel: w436 -> [_ w460]
          tunnel: w435 -> [_ w458]
          tunnel: w434 -> [_ w456]
          frame True {
            # "State is locked.  Do not run command."
          }
          frame False {
            # "Read grid"
            # "State is not locked, so may run command."
            n140 = flat-sequence {
              tunnel: [w499] -> w480
              tunnel: w454 -> [w499]
              tunnel: [w498] -> w479
              tunnel: w478 -> [w498]
              tunnel: w477 -> [w485]
              tunnel: w476 -> [w497]
              tunnel: [w497] -> w475
              tunnel: w473 -> [w496]
              tunnel: [w496] -> w474
              tunnel: [w495] -> w472
              tunnel: w471 -> [w495]
              tunnel: w470 -> [w494]
              tunnel: [w494] -> w469
              tunnel: w468 -> [w493]
              tunnel: [w493] -> w467
              tunnel: w466 -> [w492]
              tunnel: [w492] -> w465
              tunnel: w464 -> [w491]
              tunnel: [w491] -> w463
              tunnel: w462 -> [w490]
              tunnel: [w490] -> w461
              tunnel: w460 -> [w489]
              tunnel: [w489] -> w459
              tunnel: w458 -> [w488]
              tunnel: [w488] -> w457
              tunnel: w456 -> [w487]
              tunnel: [w487] -> w455
              tunnel: [w485] -> w453
              tunnel: [w521] -> w484
              tunnel: [w512] -> w483
              tunnel: w480 -> [w517]
              tunnel: w479 -> [w515]
              tunnel: w475 -> [w511]
              tunnel: w474 -> [w509]
              tunnel: w472 -> [w510]
              tunnel: w469 -> [w501]
              tunnel: w467 -> [w508]
              tunnel: w465 -> [w507]
              tunnel: w463 -> [w506]
              tunnel: w461 -> [w505]
              tunnel: w459 -> [w504]
              tunnel: w457 -> [w503]
              tunnel: w455 -> [w502]
              tunnel: w453 -> [w500]
              tunnel: w484 -> [w593]
              tunnel: w483 -> [w592]
              tunnel: [w593] -> w482
              tunnel: [w592] -> w481
              frame #0 {
                # "Prevent other commands from running."
                n141 = global write "locked.vi" "Locked"(TRUE ("Locked")) -> ()
              }
              frame #1 {
                # "Loop over each grid point"
                # "Create array\nwith grid\npoints"
                # "Close\nfile"
                # "Open file"
                n142 = Open/Create/Replace File(error in=w515, operation (0:open)=T1."replace or create with confirmation") -> (refnum out=w520:refnum<file>, error out=w514:errorcluster)  [unwired: 4 in, 1 out]
                n143 = property on="Theta axis on" class="Bool (strict)"() -> ("Value"=w516:bool)  [unwired: 2 in, 2 out]
                n144 = call "gridarray.vi"("X Start"=w505, "Y Start"=w504, "Z Start"=w503, "Theta End"=w508, "X Step"=w509, "Theta Step"=w500, "Z End"=w501, "Theta on"=w516, "Y Step"=w510, "Theta Start"=w502, "Y End"=w507, "X End"=w506, "Z Step"=w511) -> ("Array"=w522:dbl[][])  [unwired: 2 in]
                n145 = for {
                  tunnel: w522 -> [w534] mode=indexing
                  shift-right: [w525] -> w521
                  shift-left: w517 -> [w532]
                  shift-right: [w527] -> w513
                  shift-left: w514 -> [w531]
                  shift-right: [w530] -> w519
                  shift-left: w520 -> [w523]
                  tunnel: w516 -> [w529]
                  stop <- w533 stop-if-true
                  n146 = flat-sequence {
                    tunnel: w534 -> [w540]
                    tunnel: w532 -> [w548]
                    tunnel: w531 -> [w547]
                    tunnel: w529 -> [w541]
                    tunnel: [w537] -> w528
                    tunnel: [w536] -> w526
                    tunnel: [w535] -> w524
                    tunnel: w523 -> [w535]
                    tunnel: [w590] -> w530
                    tunnel: [w589] -> w527
                    tunnel: w528 -> [w567]
                    tunnel: [w566] -> w525
                    tunnel: w526 -> [w566]
                    tunnel: w524 -> [w565]
                    frame #0 {
                      # "Move to the grid point"
                      n147 = control-ref of="X pos"() -> (w549:refnum<vi>)
                      n148 = case shown="True" w541 {
                        tunnel: w540 -> [_ w555]
                        tunnel: [0.0 ("element") w554] -> w539
                        frame False {
                          # "No theta axis"
                        }
                        frame True {
                          # "Theta axis"
                          n149 = Index Array(array=w555, index=3) -> (element=w554:dbl)
                        }
                      }
                      n150 = Index Array(array=w540, index=1) -> (element=w543:dbl)
                      n151 = Index Array(array=w540, index=2) -> (element=w542:dbl)
                      n152 = Index Array(array=w540, index=0) -> (element=w544:dbl)
                      n153 = control-ref of="Z pos"() -> (w545:refnum<vi>)
                      n154 = control-ref of="Y pos"() -> (w546:refnum<vi>)
                      n155 = control-ref of="Theta pos"() -> (w538:refnum<vi>)
                      n156 = call "moveabs.vi"("Xpos"=w549, "ZPos"=w545, "YPos"=w546, "ThetaPos"=w538, "VISA resource name"=w548, "Theta on"=w541, "Y"=w543, "error in (no error)"=w547, "Z"=w542, "Theta"=w539, "X"=w544) -> ("VISA Refnum out"=w536:refnum<visa-resource-name>, "error out"=w537:errorcluster)  [unwired: 3 in]
                    }
                    frame #1 {
                      w573 = u16 1000
                      # "Write to file:\nx,y,z,theta,avgV,s.dV.,avgB,s.d.B, N"
                      # "Average"
                      # "Read voltages"
                      n157 = call "DAQ Assistant"("rate"=u16 1000, "number of samples"=w573, "error in"=w567) -> ("data"=w580:dynamicdata, "error out"=w564:errorcluster)  [unwired: 14 in, 1 out]
                      n158 = control-ref of="Theta pos"() -> (w578:refnum<vi>)
                      n159 = property class="DigNum (strict)"(reference=w578, error in=w564) -> (error out=w563:errorcluster, "Value"=w576:dbl)  [unwired: 1 out]
                      n160 = property on="Theta axis on" class="Bool (strict)"() -> ("Value"=w577:bool)  [unwired: 2 in, 2 out]
                      n161 = call "Convert from Dynamic Data"("Dynamic Data Type"=w580) -> ("Array"=w579:dbl[])  [unwired: 3 in]
                      n162 = call <vilib>:"Std Deviation and Variance.vi"("X"=w579, "Weighting (Sample)"=enum16{"Sample"}."Sample") -> ("mean"=w571:dbl, "standard deviation"=w570:dbl)  [unwired: 1 out]
                      n163 = control-ref of="Z pos"() -> (w584:refnum<vi>)
                      n164 = Select(t=w576, s=w577, f=0.0) -> (s? t:f=w574:dbl)
                      n165 = property class="DigNum (strict)"(reference=w584, error in=w563) -> (error out=w562:errorcluster, "Value"=w583:dbl)  [unwired: 1 out]
                      n166 = control-ref of="Y pos"() -> (w586:refnum<vi>)
                      n167 = property class="DigNum (strict)"(reference=w586, error in=w562) -> (error out=w561:errorcluster, "Value"=w585:dbl)  [unwired: 1 out]
                      n168 = Multiply(x=w571, y="Slope (b)") -> (x*y=w559:dbl)
                      n169 = Add(x="Intercept (a)", y=w559) -> (x+y=w572:dbl)
                      n170 = Multiply(x=w570, y="Slope (b)") -> (x*y=w569:dbl)
                      n171 = control-ref of="X pos"() -> (w588:refnum<vi>)
                      n172 = property class="DigNum (strict)"(reference=w588, error in=w561) -> (error out=w560:errorcluster, "Value"=w587:dbl)  [unwired: 1 out]
                      n173 = Format Into String(format string="%f, %f, %f, %f, %f,%f,%f, %f,%d\\n", initial string=w565, error in=w560, w587, w585, w583, w574, w571, w570, w572, w569, w573) -> (resulting string=w590:refnum<file>, error out=w589:errorcluster)
                    }
                  }
                  n174 = global read "haltnow.vi" "HaltNow"() -> (w533:bool)
                }
                n175 = Close File(refnum=w519, error in=w513) -> (error out=w512:errorcluster)  [unwired: 1 out]
              }
              frame #2 {
                # "Allow other commands to run."
                n176 = global write "locked.vi" "Locked"(FALSE ("Locked")) -> ()
              }
            }
          }
        }
      }
      frame 32 {
        # "Clear VISA buffers"
        n177 = VISA Clear(VISA resource name=w597, error in (no error)=w596) -> (VISA resource name out=w595:refnum<visa-resource-name>, error out=w594:errorcluster)
      }
    }
  }
  n178 = VISA Close(VISA resource name=w1, error in (no error)=w2) -> (error out=w5:errorcluster)
  n179 = call <vilib>:"Simple Error Handler.vi"("error in (no error)"=w5) -> ("message"=→"message":string)  [unwired: 4 in, 4 out]
